vi "compute path cluster.vi"(2 "path queue":refnum<queue>, 3 "Arrive simultaeously":bool, 4 "error in (no error)":errorcluster, 5 "Step length\n(IMAQ pixels)":dbl, 7 "waypoint queue":refnum<queue>) -> (0 "error out":errorcluster)   [LabVIEW 2011]
uses:
  Trap cluster.ctl
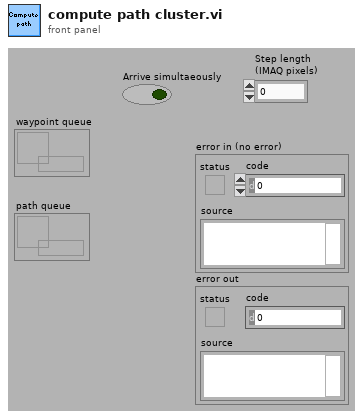
[diagram p1: front panel]
types:
  T1 = typedef "Trap cluster.ctl" = cluster{"X (IMAQ)":sgl[], "Y (IMAQ)":sgl[], "Z":sgl[], "I":sgl[], "Trap number":i32[], "ROI number":i32[], "Number of traps":i32, "Group":bool[]}
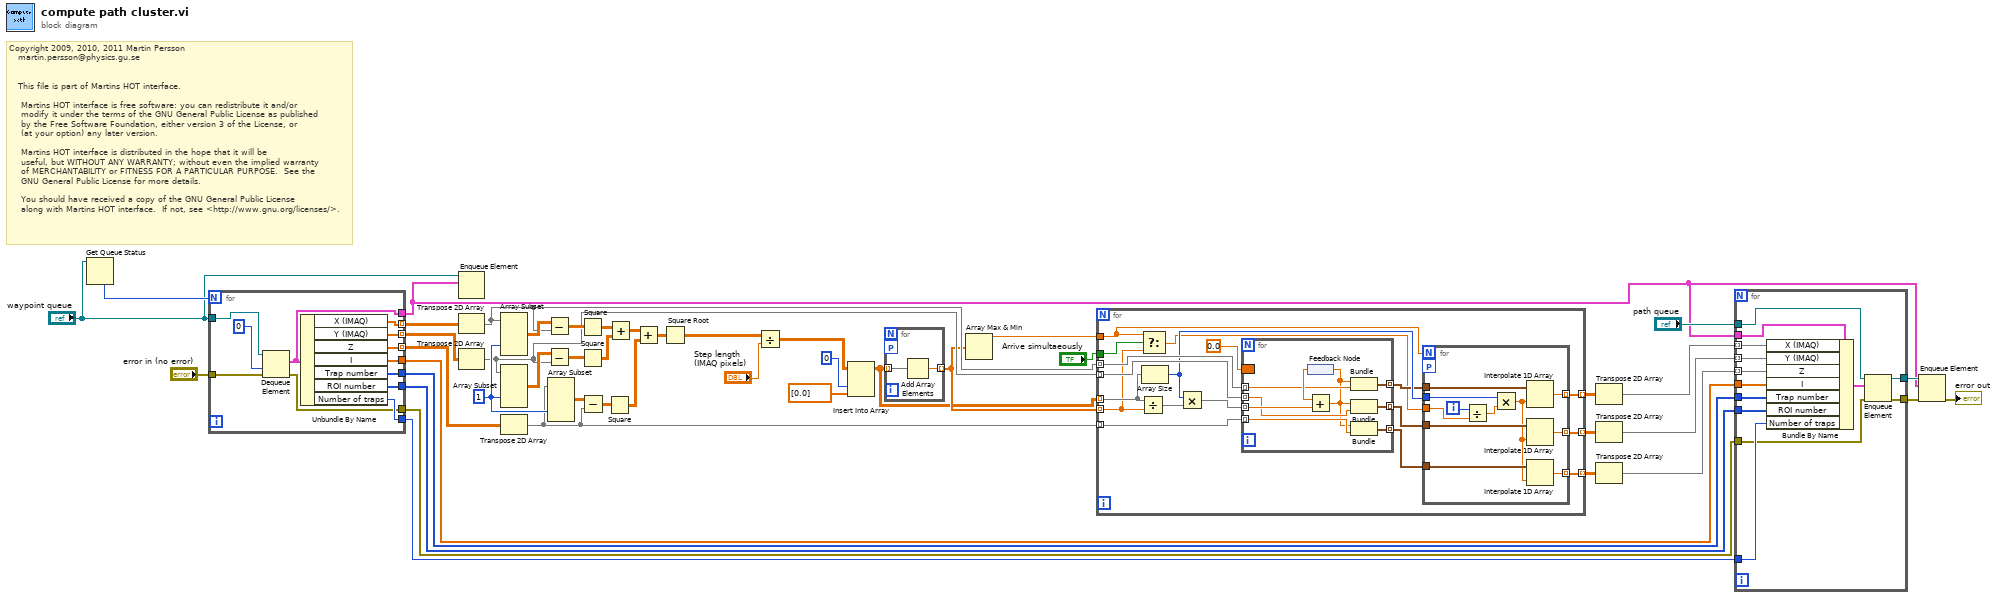
[diagram p0: block diagram]
diagram:
  w43 = 1 ("index")
  # "Copyright 2009, 2010, 2011 Martin Persson \n   martin.persson@physics.gu.se\n\n\n   This file is part of Martins HOT interface.\n\n    Martins HOT interface is free software: you can redistribute it and/or \n    modify it under the terms of the GNU General Public License as published \n    by the Free Software Foundation, either version 3 of the License, or\n    (at your option) any later version.\n\n    Martins HOT interface is distributed in the hope that it will be \n    useful, but WITHOUT ANY WARRANTY; without even the implied warranty\n    of MERCHANTABILITY or FITNESS FOR A PARTICULAR PURPOSE.  See the\n    GNU General Public License for more details.\n\n    You should have received a copy of the GNU General Public License\n    along with Martins HOT interface.  If not, see <http://www.gnu.org/licenses/>."
  n1 = Get Queue Status(queue="waypoint queue") -> (# elements in queue=w6:i32)  [unwired: 2 in, 7 out]
  n2 = for {
    N: w6 -> [_]
    tunnel: [w58] -> w46 mode=indexing
    tunnel: [w57] -> w45 mode=indexing
    tunnel: [w56] -> w44 mode=indexing
    tunnel: [w55] -> w13
    tunnel: [w54] -> w12
    tunnel: [w53] -> w11
    tunnel: [w52] -> w10
    tunnel: [w51] -> w3
    tunnel: "waypoint queue" -> [w50]
    tunnel: "error in (no error)" -> [w49]
    tunnel: [w48] -> w7
    n3 = Dequeue Element(queue=w50, timeout in ms (-1)=0, error in (no error)=w49) -> (element=w51:T1, error out=w48:errorcluster)  [unwired: 2 out]
    n4 = Unbundle By Name(w51) -> ("X (IMAQ)"=w58:sgl[], "Y (IMAQ)"=w57:sgl[], "Z"=w56:sgl[], "I"=w55:sgl[], "Trap number"=w54:i32[], "ROI number"=w53:i32[], "Number of traps"=w52:i32)
  }
  n5 = Enqueue Element(queue="waypoint queue", element=w3) -> ()  [unwired: 2 in, 3 out]
  n6 = Transpose 2D Array(2D array=w46) -> (transposed array=w27:sgl[][])
  n7 = Transpose 2D Array(2D array=w45) -> (transposed array=w26:sgl[][])
  n8 = Array Subset(array=w27, index (col)=w43) -> (w32:sgl[][])  [unwired: 3 in]
  n9 = Array Subset(array=w26, index (col)=w43) -> (w31:sgl[][])  [unwired: 3 in]
  n10 = Transpose 2D Array(2D array=w44) -> (transposed array=w25:sgl[][])
  n11 = Subtract(x=w32, y=w27) -> (x-y=w42:sgl[][])
  n12 = Subtract(x=w31, y=w26) -> (x-y=w41:sgl[][])
  n13 = Array Subset(array=w25, index (col)=w43) -> (w30:sgl[][])  [unwired: 3 in]
  n14 = Square(x=w42) -> (x^2=w39:sgl[][])
  n15 = Square(x=w41) -> (x^2=w38:sgl[][])
  n16 = Subtract(x=w30, y=w25) -> (x-y=w40:sgl[][])
  n17 = Square(x=w40) -> (x^2=w36:sgl[][])
  n18 = Add(x=w39, y=w38) -> (x+y=w37:sgl[][])
  n19 = Add(x=w37, y=w36) -> (x+y=w35:sgl[][])
  n20 = Square Root(x=w35) -> (sqrt(x)=w34:sgl[][])
  n21 = Divide(x=w34, y="Step length\n(IMAQ pixels)") -> (x/y=w22:dbl[][])
  n22 = Insert Into Array(array=w22, index (col)=0 ("disabled index (col)"), new element=dbl[] [0.0] ("new element/subarray")) -> (w21:dbl[][])  [unwired: 1 in]
  n23 = for {
    tunnel: w21 -> [w60] mode=indexing
    tunnel: [w59] -> w23 mode=indexing
    workers-P: _ -> [_]
    n24 = Add Array Elements(numeric array=w60) -> (sum=w59:dbl)
  }
  n25 = Array Max & Min(array=w23) -> (max value=w24:dbl)  [unwired: 3 out]
  n26 = for {
    tunnel: w21 -> [w76] mode=indexing
    tunnel: w27 -> [w74] mode=indexing
    tunnel: w26 -> [w73] mode=indexing
    tunnel: w25 -> [w72] mode=indexing
    tunnel: w24 -> [w62]
    tunnel: [w69] -> w19 mode=indexing
    tunnel: w23 -> [w63] mode=indexing
    tunnel: [w66] -> w18 mode=indexing
    tunnel: [w65] -> w17 mode=indexing
    tunnel: "Arrive simultaeously" -> [w61]
    n27 = Divide(x=w76, y=w63) -> (x/y=w78:dbl[])
    n28 = Select(t=w62, s=w61, f=w63) -> (s? t:f=w64:dbl)
    n29 = Array Size(array=w76) -> (size(s)=w71:i32)
    n30 = Multiply(x=w71, y=w78) -> (x*y=w75:dbl[])
    n31 = for {
      tunnel: w75 -> [w98] mode=indexing
      border: 0.0 -> [_]
      tunnel: w74 -> [w96] mode=indexing
      tunnel: w73 -> [w95] mode=indexing
      tunnel: w72 -> [w94] mode=indexing
      tunnel: [w92] -> w70 mode=indexing
      tunnel: [w91] -> w68 mode=indexing
      tunnel: [w90] -> w67 mode=indexing
      n32 = feedback #1() -> (w97:dbl)
      n33 = Add(x=w97, y=w98) -> (x+y=w93:dbl)
      n34 = feedback-in #1(w93) -> ()
      n35 = Bundle(w93, w96) -> (w92:cluster{dbl, sgl})  [unwired: 1 in]
      n36 = Bundle(w93, w95) -> (w91:cluster{dbl, sgl})  [unwired: 1 in]
      n37 = Bundle(w93, w94) -> (w90:cluster{dbl, sgl})  [unwired: 1 in]
    }
    n38 = for {
      N: w62 -> [_]
      tunnel: w64 -> [w88]
      tunnel: w71 -> [w86]
      tunnel: w70 -> [w85]
      tunnel: [w84] -> w69 mode=indexing
      tunnel: w68 -> [w83]
      tunnel: w67 -> [w82]
      tunnel: [w80] -> w66 mode=indexing
      tunnel: [w79] -> w65 mode=indexing
      workers-P: _ -> [_]
      i -> [w89]
      n39 = Divide(x=w89, y=w88) -> (x/y=w87:dbl)
      n40 = Multiply(x=w86, y=w87) -> (x*y=w81:dbl)
      n41 = Interpolate 1D Array(1:w81, 2:w85) -> (0:w84:sgl)
      n42 = Interpolate 1D Array(1:w81, 2:w83) -> (0:w80:sgl)
      n43 = Interpolate 1D Array(1:w81, 2:w82) -> (0:w79:sgl)
    }
  }
  n44 = Transpose 2D Array(2D array=w19) -> (transposed array=w16:sgl[][])
  n45 = Transpose 2D Array(2D array=w18) -> (transposed array=w15:sgl[][])
  n46 = Transpose 2D Array(2D array=w17) -> (transposed array=w14:sgl[][])
  n47 = for {
    tunnel: w16 -> [w111] mode=indexing
    tunnel: w15 -> [w110] mode=indexing
    tunnel: w14 -> [w109] mode=indexing
    tunnel: w13 -> [w108]
    tunnel: w12 -> [w107]
    tunnel: w11 -> [w106]
    tunnel: w10 -> [w105]
    tunnel: w3 -> [w104]
    tunnel: "path queue" -> [w103]
    tunnel: w7 -> [w102]
    tunnel: [w101] -> w2
    tunnel: [w99] -> w4
    n48 = Bundle By Name(cluster=w104, "X (IMAQ)"=w111, "Y (IMAQ)"=w110, "Z"=w109, "I"=w108, "Trap number"=w107, "ROI number"=w106, "Number of traps"=w105) -> (w100:T1)
    n49 = Enqueue Element(queue=w103, element=w100, error in (no error)=w102) -> (queue out=w99:refnum<queue>, error out=w101:errorcluster)  [unwired: 1 in, 1 out]
  }
  n50 = Enqueue Element(queue=w4, element=w3, error in (no error)=w2) -> (error out=→"error out":errorcluster)  [unwired: 1 in, 2 out]
